vi "Main Page.vi"(8 "error in (no error)":errorcluster, 11 "Node Ptr":T7 format="%.0x") -> (0 "error out":errorcluster)   [LabVIEW 2015, in "Modbus Master System Explorer.lvlib"]
uses:
  Modbus Master System Explorer.lvlib
  <vilib>/NI Veristand/Custom Device API/Custom Device Item Ref.ctl
  Shared/Controls/Interface Type.ctl
  Shared/Controls/Parity.ctl
  Shared/Controls/Serial Type.ctl
  Shared/Controls/Flow Control.ctl
  SubVIs/Radix.ctl
  Shared/Constants.vi
  <vilib>/NI Veristand/Custom Device API/Set Item Property (U16).vi
  <vilib>/NI VeriStand/Custom Device API/Custom Device API.lvlib
  Shared/Modbus Master Shared.lvlib
panel:
  in  "WebBrowser":refnum<k7>(container)
  in  "Maximum Channels per Read":i32
  in  "Read Refresh Rate (ms)":i32
  in  "Export to Kepware Server":bool
  in  "Name":string
  in  "Master Settings Tabs":enum32{"TCP Master", "Serial Master"}(tab)
  in  "Timeout (ms)":i32
  in  "Address":string
  in  "Port":u16
  in  "Wire Mode":T1(ring)
  in  "Baud Rate":string(combo)
  in  "Radix":T2
  in  "Unit ID":u16
  out "Data Bits":u32=7
  in  "VISA resource name":refnum<visa-resource-name>
  in  "flow control (none)":T3 items=["None", "XON/XOFF", "RTS/CTS", "XON/XOFF & RTS/CTS", "DTR/DSR", "XON/XOFF & DTR/DSR"]
  in  "parity (even)":T4=2 items=["None", "Odd", "Even", "Mark", "Space"]
  in  "serial type":T5
  out "Stop Bits":u32
  in  "Interface Type":T6
  in  "Header":cluster{"Section Name":string}={"Section Name"="Modbus Master to Slave Settings"}
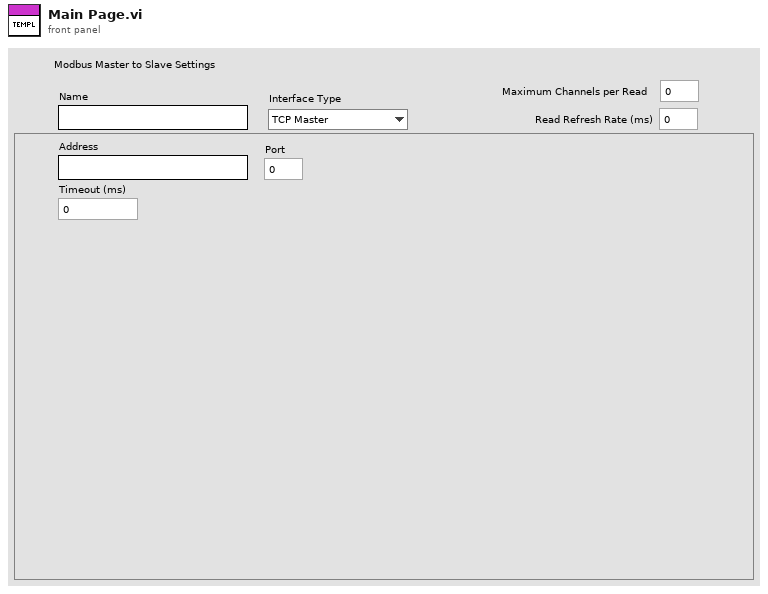
[diagram p1: front panel]
types:
  T1 = enum16{"Unknown", "RS485/Wire4", "RS485/Wire2-EchoDTR", "RS485/Wire2-CtrlDTR", "RS485/Wire2-Auto", "RS232/DTE", "RS232/DCE", "RS232/AUTO"}
  T2 = typedef "Modbus Master System Explorer.lvlib/Radix.ctl" = enum32{"Decimal", "Hexidecimal"}
  T3 = typedef "Modbus Master Shared.lvlib/Flow Control.ctl" = u16
  T4 = typedef "Modbus Master Shared.lvlib/Parity.ctl" = u16
  T5 = typedef "Modbus Master Shared.lvlib/Serial Type.ctl" = enum16{"RTU", "ASCII"}
  T6 = typedef "Modbus Master Shared.lvlib/Interface Type.ctl" = enum16{"TCP Master", "Serial Master", "TCP Slave", "Serial Slave"}
  T7 = typedef "Custom Device API.lvlib/Custom Device Item Ref.ctl" = u64
  T8 = typedef "Custom Device API.lvlib/Custom Device Commands.ctl" = enum16{"Default", "Item renamed", "Shutdown", "Dynamic button pressed"}
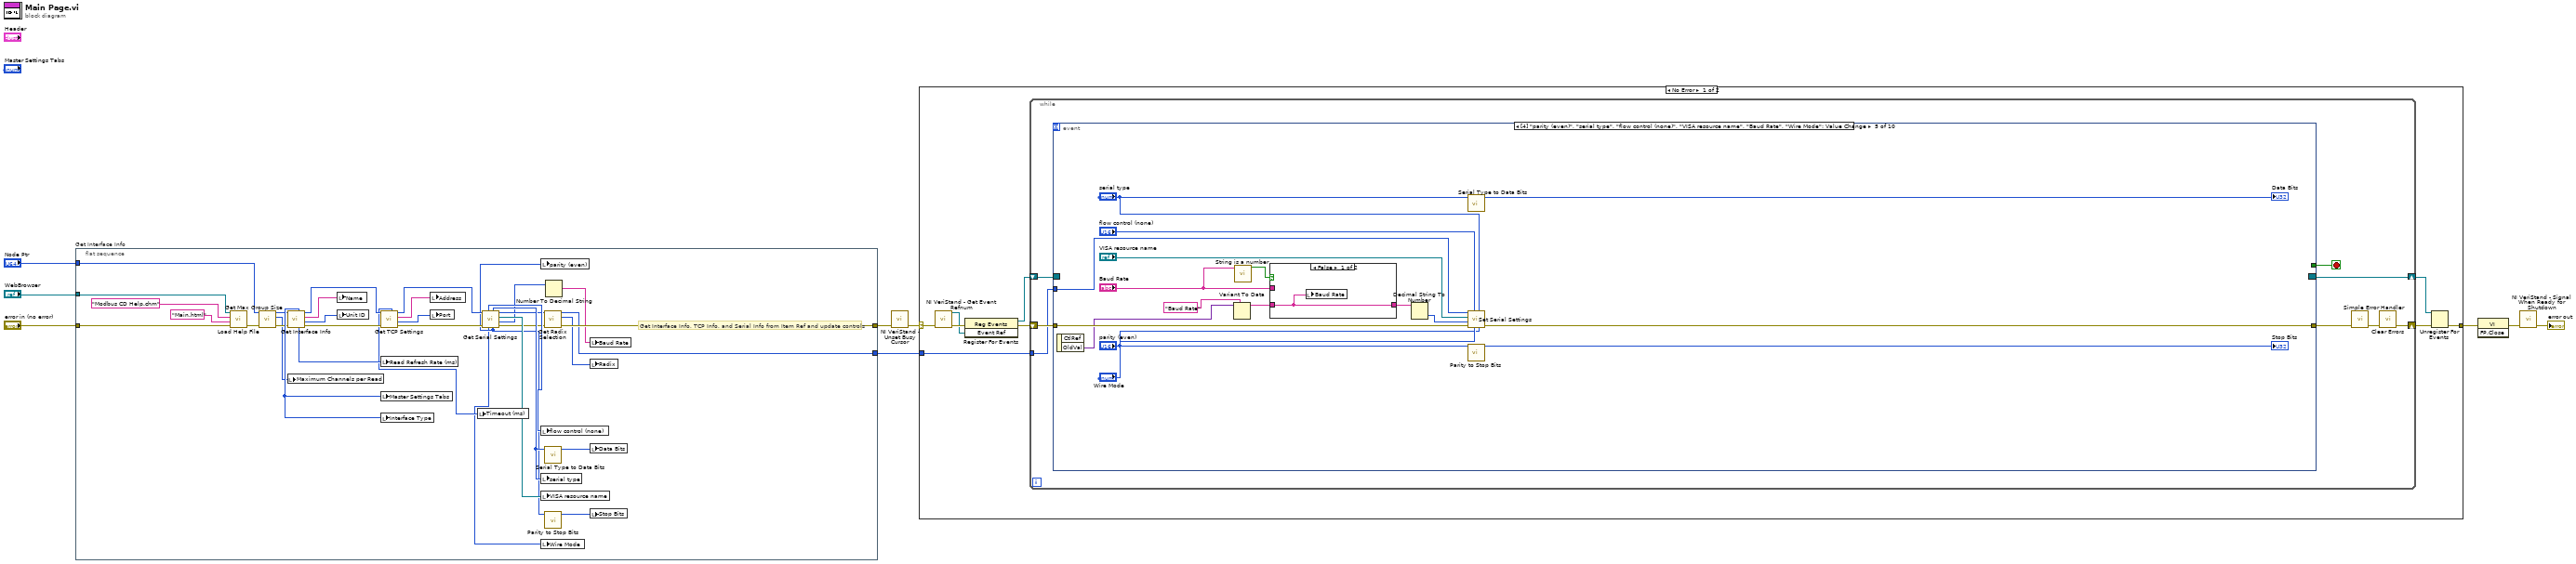
[diagram p0: block diagram]
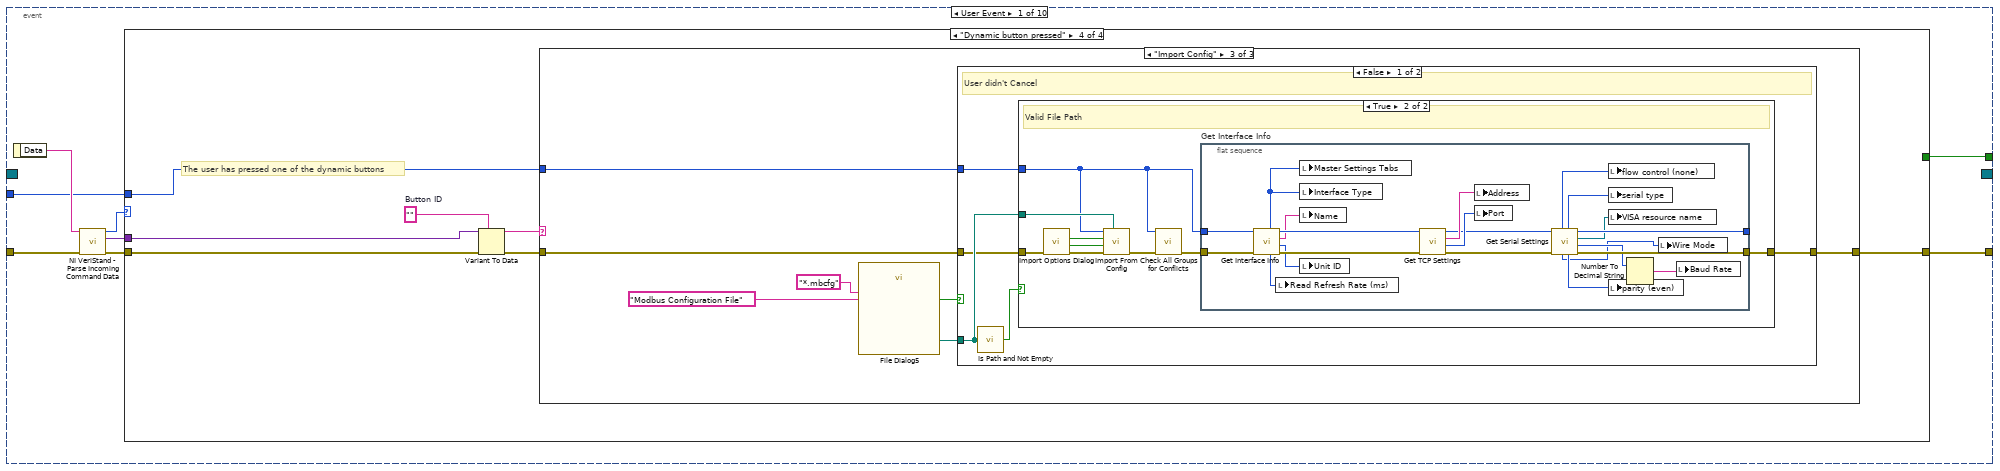
[diagram p2: hidden frame]
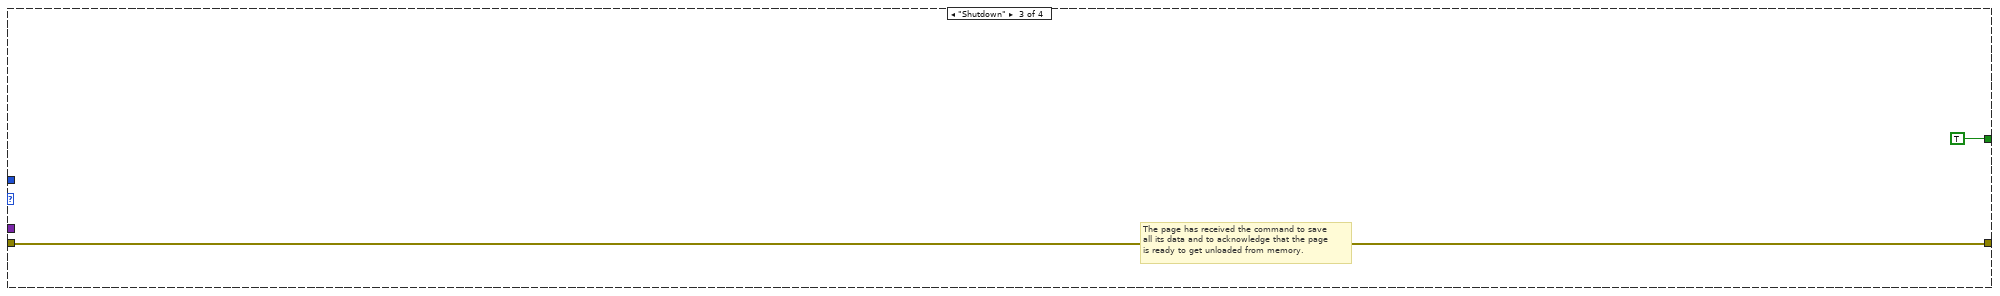
[diagram p5: hidden frame]
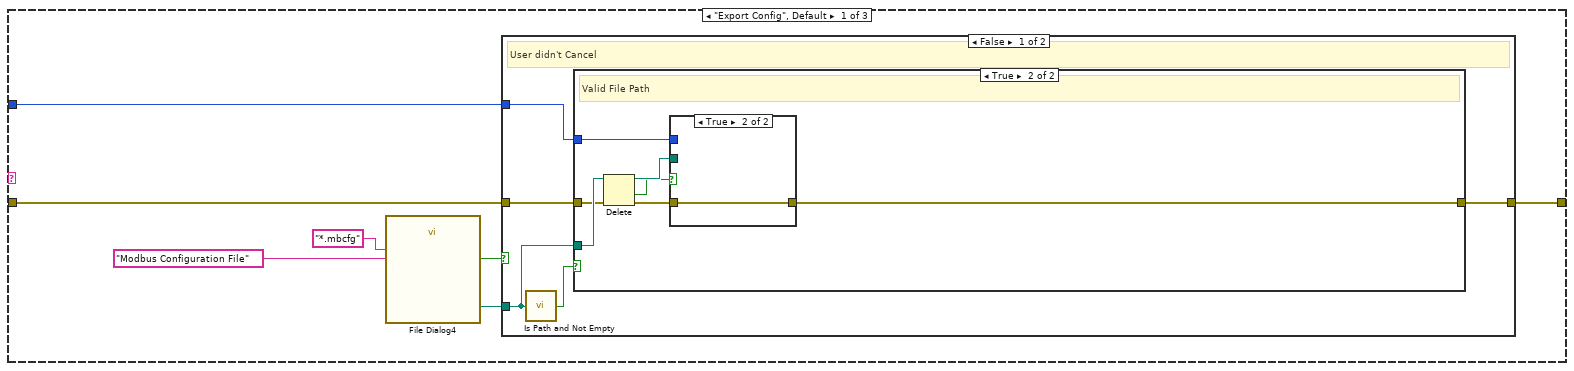
[diagram p6: hidden frame]
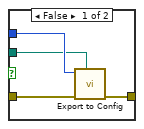
[diagram p8: hidden frame]
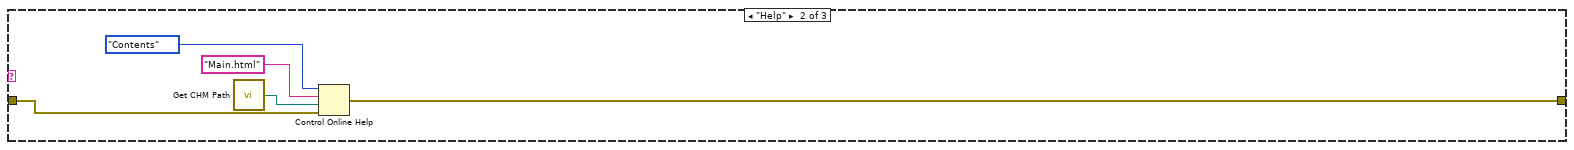
[diagram p10: hidden frame]
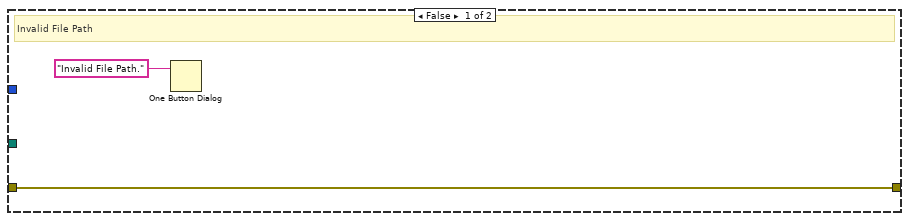
[diagram p11: hidden frame]
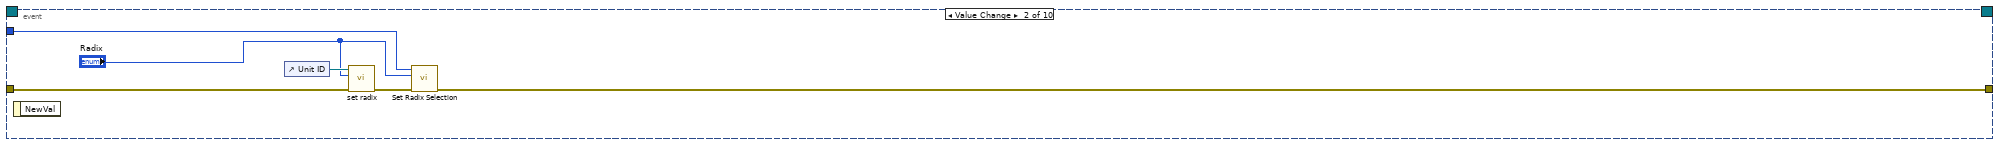
[diagram p13: hidden frame]
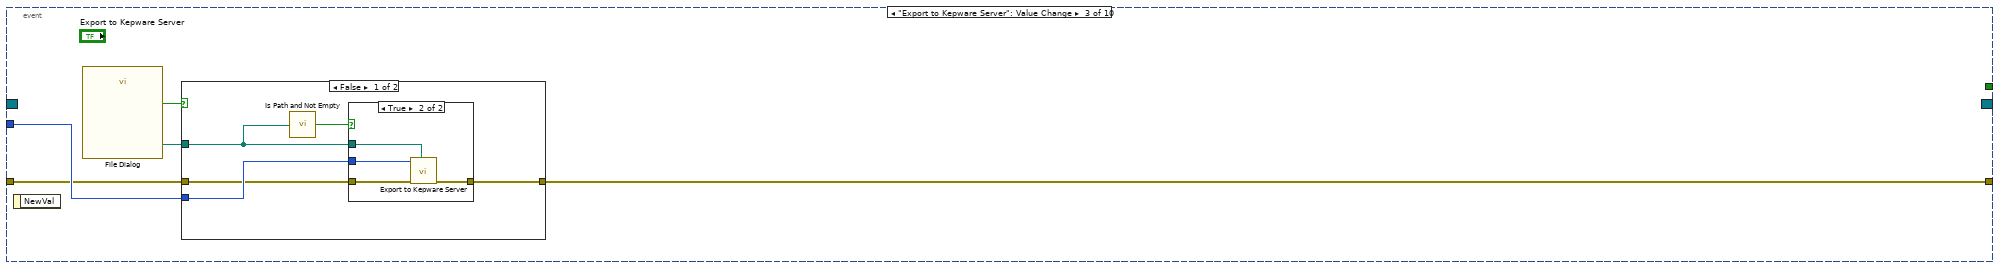
[diagram p14: hidden frame]
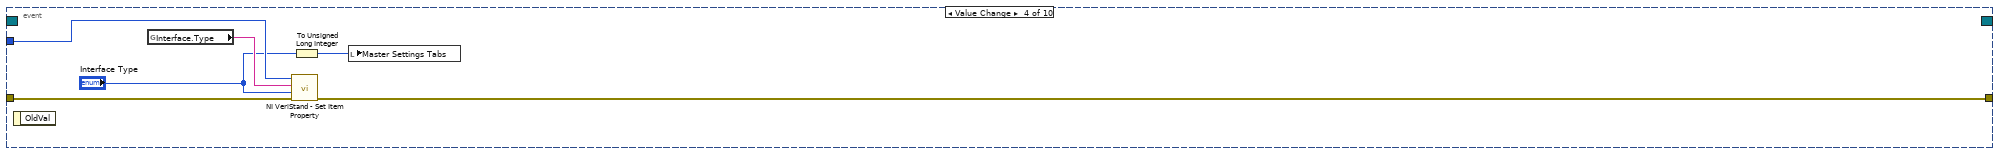
[diagram p17: hidden frame]
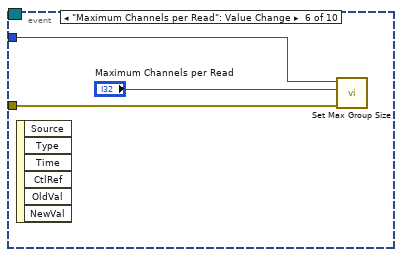
[diagram p19: hidden frame]
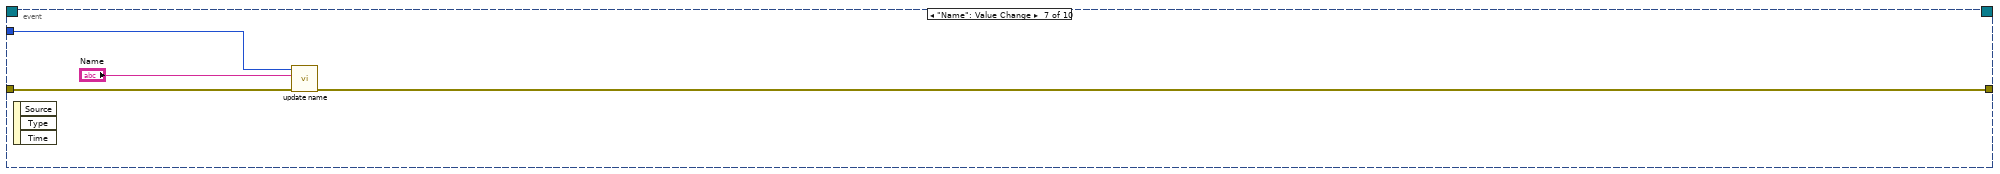
[diagram p20: hidden frame]
diagram:
  n1 = flat-sequence "Get Interface Info" {
    tunnel: "error in (no error)" -> [w12]
    tunnel: "Node Ptr" -> [w27]
    tunnel: [w21] -> w3
    tunnel: [w19] -> w2
    tunnel: "WebBrowser" -> [w15]
    frame #0 {
      # "Get Interface Info, TCP Info, and Serial Info from Item Ref and update controls"
      n2 = call "Load Help File.vi"("error in (no error)"=w12, "HTML File"="Main.html", "Main CHM File"="Modbus CD Help.chm", "SHDocVw.IWebBrowser2"=w15) -> ("error out"=w11:errorcluster)  [unwired: 7 in]
      n3 = call "Get Max Group Size.vi"("error in (no error)"=w11, "Item Ref in"=w27) -> ("error out"=w25:errorcluster, "Value"=w24:i32, "Item Ref out"=w26:T7)  [unwired: 7 in]
      n4 = call "Get Interface Info.vi"("error in (no error)"=w25, "Device Item Ref in"=w26) -> ("error out"=w36:errorcluster, "Unit ID"=w33:u16, "Name"=w34:string, "Item Ref out"=w37:T7, "Refresh Rate"=w32:i32, "Interface Type"=w35:T6)  [unwired: 4 in]
      n5 = local write "Maximum Channels per Read"(w24) -> ()
      n6 = local write "Name"(w34) -> ()
      n7 = local write "Unit ID"(w33) -> ()
      n8 = call "Get TCP Settings.vi"("error in (no error)"=w36, "Item Ref in"=w37) -> ("error out"=w41:errorcluster, "Port"=w42:u16, "Address"=w43:string, "Item Ref out"=w40:T7, "Timeout"=w23:i32)  [unwired: 5 in]
      n9 = local write "Read Refresh Rate (ms)"(w32) -> ()
      n10 = local write "Master Settings Tabs"(w35) -> ()
      n11 = local write "Interface Type"(w35) -> ()
      n12 = local write "Address"(w43) -> ()
      n13 = local write "Port"(w42) -> ()
      n14 = local write "Timeout (ms)"(w23) -> ()
      n15 = call "Get Serial Settings.vi"("error in (no error)"=w41, "Item Ref in"=w40) -> ("error out"=w22:errorcluster, "baud rate"=w17:u32, "VISA resource name"=w38:refnum<visa-resource-name>, "Item Ref out"=w20:T7, "parity (even)"=w29:T4, "serial type"=w30:T5, "Wire Mode"=w10:i16, "flow control (none)"=w39:T3)  [unwired: 2 in]
      n16 = local write "parity (even)"(w29) -> ()
      n17 = local write "flow control (none)"(w39) -> ()
      n18 = local write "serial type"(w30) -> ()
      n19 = local write "VISA resource name"(w38) -> ()
      n20 = local write "Wire Mode"(w10) -> ()
      n21 = call "Get Radix Selection.vi"("error in (no error)"=w22, "Item Ref in"=w20) -> ("error out"=w21:errorcluster, "Radix"=w18:T2, "Item Ref out"=w19:T7)  [unwired: 7 in]
      n22 = call "Serial Type to Data Bits.vi"("serial type"=w30) -> ("Data Bits"=w31:u32)  [unwired: 10 in]
      n23 = call "Parity to Stop Bits.vi"("parity"=w29) -> ("Stop Bits"=w28:u32)  [unwired: 10 in]
      n24 = Number To Decimal String(number=w17) -> (decimal integer string=w16:string)  [unwired: 1 in]
      n25 = local write "Baud Rate"(w16) -> ()
      n26 = local write "Radix"(w18) -> ()
      n27 = local write "Data Bits"(w31) -> ()
      n28 = local write "Stop Bits"(w28) -> ()
    }
  }
  n29 = call <vilib>:"NI VeriStand - Unset Busy Cursor.vi"("error in (no error)"=w3) -> ("error out"=w5:errorcluster)  [unwired: 10 out]
  n30 = case shown="No Error" w5 {
    selector: w5 -> [w44 w227]
    tunnel: [w49 w225] -> w9
    tunnel: w2 -> [w45 _]
    frame No Error {
      n31 = call <vilib>:"NI VeriStand - Get Event Refnum.vi"("error in (no error)"=w44) -> ("error out"=w52:errorcluster, "Event Ref"=w48:refnum<user-event>)  [unwired: 9 out]
      n32 = register-events(error in=w52, w48) -> (reference out=w46:refnum<event-registration>, error out=w47:errorcluster)  [unwired: 1 in]
      n33 = while {
        tunnel: w45 -> [w56]
        shift-right: [w53] -> w50
        shift-left: w47 -> [w59]
        shift-right: [w60] -> w51
        shift-left: w46 -> [w58]
        stop <- w57 stop-if-true
        n34 = event shown="[4] \"parity (even)\", \"serial type\", \"flow control (none)\", \"VISA resource name\", \"Baud Rate\", \"Wire Mode\": Value Change" {
          selector: w58 -> [_ _ _ _ _ _ _ _ _ _]
          dyn-events: [_ _ _ _ _ _ _ _ _ _] -> w60
          timeout: _ -> [_ _ _ _ _ _ _ _ _ _]
          tunnel: w59 -> [w68 w159 w163 w181 w198 w203 w207 w211 w217 w223]
          tunnel: [w64 _ _ _ _ _ _ _ _ _] -> w57
          tunnel: [w63 w157 w162 w178 w196 _ w206 w210 w216 w222] -> w55
          tunnel: w56 -> [w62 w161 w164 w182 w199 w205 w209 w212 w218 w224]
          event User Event {
            n35 = event-data() -> ("Data"=w67:string)  [unwired: 1 out]
            n36 = call <vilib>:"NI VeriStand - Parse Incoming Command Data.vi"("error in (no error)"=w68, "Incoming data"=w67) -> ("error out"=w66:errorcluster, "Outgoing data"=w61:variant, "Action"=w65:T8)  [unwired: 7 out]
            n37 = case shown="\"Dynamic button pressed\"" w65 {
              tunnel: w66 -> [w69 w70 w71 w79]
              tunnel: [_ _ TRUE _] -> w64
              tunnel: [w69 w70 w71 w73] -> w63
              tunnel: w62 -> [_ _ _ w75]
              tunnel: w61 -> [_ _ _ w78]
              frame "Default", Default {
              }
              frame "Item renamed" {
              }
              frame "Shutdown" {
                # "The page has received the command to save all its data and to acknowledge that the page is ready to get unloaded from memory."
              }
              frame "Dynamic button pressed" {
                w77 = ""  # Button ID
                # "The user has pressed one of the dynamic buttons"
                n38 = Variant To Data(error in=w79, type=w77, Variant=w78) -> (data=w76:string, error out=w74:errorcluster)
                n39 = case shown="\"Import Config\"" w76 {
                  tunnel: w75 -> [w84 _ w115]
                  tunnel: w74 -> [w83 w107 w114]
                  tunnel: [w82 w106 w113] -> w73
                  frame "Export Config", Default {
                    n40 = call "File Dialog4"("pattern (all files)"="*.mbcfg", "pattern label"="Modbus Configuration File") -> ("selected path"=w86:path, "cancelled"=w85:bool)  [unwired: 10 in, 2 out]
                    n41 = case shown="False" w85 {
                      tunnel: w86 -> [w90 _]
                      tunnel: w84 -> [w89 _]
                      tunnel: w83 -> [w88 w105]
                      tunnel: [w87 w105] -> w82
                      frame False {
                        # "User didn't Cancel"
                        n42 = call <vilib>:"Is Path and Not Empty.vi"("path"=w90) -> ("Is Path and Not Empty?"=w91:bool)  [unwired: 4 in]
                        n43 = case shown="True" w91 {
                          tunnel: w90 -> [_ w97]
                          tunnel: w89 -> [_ w98]
                          tunnel: w88 -> [w92 w94]
                          tunnel: [w92 w99] -> w87
                          frame False {
                          }
                          frame True {
                            # "Valid File Path"
                            n44 = Delete(path (use dialog)=w97, error in=w94) -> (deleted path=w96:path, cancelled=w95:bool, error out=w93:errorcluster)  [unwired: 3 in]
                            n45 = case shown="True" w95 {
                              tunnel: w93 -> [w103 w104]
                              tunnel: [w102 w104] -> w99
                              tunnel: w98 -> [w101 _]
                              tunnel: w96 -> [w100 _]
                              frame False {
                                n46 = call "Export to Config.vi"("selected path"=w100, "error in"=w103, "Device Ref in"=w101) -> ("error out"=w102:errorcluster)  [unwired: 8 in]
                              }
                              frame True {
                              }
                            }
                          }
                        }
                      }
                      frame True {
                      }
                    }
                  }
                  frame "Help" {
                    n47 = call "Get CHM Path.vi"() -> ("appended path"=w110:path)
                    n48 = Control Online Help(1:w107, 2:w110, 3:"Main.html" ("String to search for"), 4:enum16{"Contents", "Key", "Close"}."Contents" ("Operation")) -> (0:w106:errorcluster)
                  }
                  frame "Import Config" {
                    n49 = call "File Dialog5"("pattern (all files)"="*.mbcfg", "pattern label"="Modbus Configuration File") -> ("selected path"=w117:path, "cancelled"=w116:bool)  [unwired: 10 in, 2 out]
                    n50 = case shown="False" w116 {
                      tunnel: w117 -> [w121 _]
                      tunnel: w115 -> [w120 _]
                      tunnel: w114 -> [w119 w155]
                      tunnel: [w118 w155] -> w113
                      frame False {
                        # "User didn't Cancel"
                        n51 = call <vilib>:"Is Path and Not Empty.vi"("path"=w121) -> ("Is Path and Not Empty?"=w122:bool)  [unwired: 4 in]
                        n52 = case shown="True" w122 {
                          tunnel: w121 -> [_ w133]
                          tunnel: w120 -> [_ w131]
                          tunnel: w119 -> [w124 w128]
                          tunnel: [w124 w129] -> w118
                          frame False {
                            # "Invalid File Path"
                            n53 = One Button Dialog(message="Invalid File Path.") -> ()  [unwired: 1 in, 1 out]
                          }
                          frame True {
                            # "Valid File Path"
                            n54 = call "Import Options Dialog.vi"("error in (no error)"=w128) -> ("error out"=w127:errorcluster, "Overwrite Existing Channels?"=w125:bool, "Overwrite Device Settings?"=w126:bool)  [unwired: 8 in]
                            n55 = call "Import From Config.vi"("selected path"=w133, "error in"=w127, "Overwrite Existing Channels?"=w125, "Overwrite Device Settings?"=w126, "Device Ref in"=w131) -> ("error out"=w132:errorcluster)  [unwired: 6 in]
                            n56 = call "Check All Groups for Conflicts.vi"("error in (no error)"=w132, "Item Ref in"=w131) -> ("error out"=w130:errorcluster)  [unwired: 9 in]
                            n57 = flat-sequence "Get Interface Info" {
                              tunnel: w130 -> [w137]
                              tunnel: w131 -> [w138]
                              tunnel: [w151] -> w129
                              tunnel: [w149] -> _
                              frame #0 {
                                n58 = call "Get Interface Info.vi"("error in (no error)"=w137, "Device Item Ref in"=w138) -> ("error out"=w143:errorcluster, "Unit ID"=w140:u16, "Name"=w141:string, "Item Ref out"=w144:T7, "Refresh Rate"=w139:i32, "Interface Type"=w142:T6)  [unwired: 4 in]
                                n59 = local write "Read Refresh Rate (ms)"(w139) -> ()
                                n60 = local write "Master Settings Tabs"(w142) -> ()
                                n61 = local write "Interface Type"(w142) -> ()
                                n62 = local write "Name"(w141) -> ()
                                n63 = local write "Unit ID"(w140) -> ()
                                n64 = call "Get TCP Settings.vi"("error in (no error)"=w143, "Item Ref in"=w144) -> ("error out"=w152:errorcluster, "Port"=w153:u16, "Address"=w154:string, "Item Ref out"=w150:T7)  [unwired: 5 in, 1 out]
                                n65 = local write "Address"(w154) -> ()
                                n66 = local write "Port"(w153) -> ()
                                n67 = call "Get Serial Settings.vi"("error in (no error)"=w152, "Item Ref in"=w150) -> ("error out"=w151:errorcluster, "baud rate"=w136:u32, "VISA resource name"=w145:refnum<visa-resource-name>, "Item Ref out"=w149:T7, "parity (even)"=w148:T4, "serial type"=w147:T5, "Wire Mode"=w134:i16, "flow control (none)"=w146:T3)  [unwired: 2 in]
                                n68 = local write "flow control (none)"(w146) -> ()
                                n69 = local write "serial type"(w147) -> ()
                                n70 = local write "VISA resource name"(w145) -> ()
                                n71 = local write "parity (even)"(w148) -> ()
                                n72 = Number To Decimal String(number=w136) -> (decimal integer string=w135:string)  [unwired: 1 in]
                                n73 = local write "Wire Mode"(w134) -> ()
                                n74 = local write "Baud Rate"(w135) -> ()
                              }
                            }
                          }
                        }
                      }
                      frame True {
                        # "User Canecelled, do nothing"
                      }
                    }
                  }
                }
              }
            }
          }
          event Value Change {
            n75 = event-data() -> ()  [unwired: 2 out]
            n76 = control-ref of="Unit ID"() -> (w160:refnum<vi>)
            n77 = call "set radix.vi"("error in (no error)"=w159, "Radix"="Radix", "Digital in"=w160) -> ("error out"=w158:errorcluster)  [unwired: 8 in]
            n78 = call "Set Radix Selection.vi"("error in (no error)"=w158, "Radix"="Radix", "Item Ref in"=w161) -> ("error out"=w157:errorcluster)  [unwired: 7 in, 1 out]
          }
          event "Export to Kepware Server": Value Change {
            n79 = event-data() -> ()  [unwired: 2 out]
            n80 = call "File Dialog"() -> ("selected path"=w166:path, "cancelled"=w165:bool)  [unwired: 12 in, 2 out]
            n81 = case shown="False" w165 {
              tunnel: w166 -> [w170 _]
              tunnel: w164 -> [w169 _]
              tunnel: w163 -> [w168 w177]
              tunnel: [w167 w177] -> w162
              frame False {
                n82 = call <vilib>:"Is Path and Not Empty.vi"("path"=w170) -> ("Is Path and Not Empty?"=w171:bool)  [unwired: 4 in]
                n83 = case shown="True" w171 {
                  tunnel: w170 -> [_ w176]
                  tunnel: w169 -> [_ w175]
                  tunnel: w168 -> [w172 w174]
                  tunnel: [w172 w173] -> w167
                  frame False {
                  }
                  frame True {
                    n84 = call "Export to Kepware Server.vi"("selected path"=w176, "error in"=w174, "Device Ref in"=w175) -> ("error out"=w173:errorcluster)  [unwired: 8 in]
                  }
                }
              }
              frame True {
              }
            }
          }
          event Value Change {
            n85 = event-data() -> ()  [unwired: 2 out]
            n86 = global read "Constants.vi" "Interface.Type"() -> (w183:string)
            n87 = call-poly <vilib>:"NI VeriStand - Set Item Property.vi"("error in (no error)"=w181, "Value"="Interface Type", "Property Name"=w183, "Item Ref in"=w182) -> ("error out"=w178:errorcluster)  [unwired: 5 in, 2 out]
            n88 = To Unsigned Long Integer(number="Interface Type") -> (unsigned 32bit integer=w180:u32)
            n89 = local write "Master Settings Tabs"(w180) -> ()
          }
          event "VISA resource name", "Baud Rate", "Wire Mode": Value Change {
            n90 = event-data() -> ("OldVal"=w186:variant)  [unwired: 2 out]
            n91 = Variant To Data(type="Baud Rate" ("y"), Variant=w186) -> (data=w185:string)  [unwired: 1 in, 1 out]
            n92 = call "String is a number.vi"("Baud Rate"="Baud Rate") -> ("Boolean"=w189:bool)  [unwired: 10 in]
            n93 = case shown="False" w189 {
              tunnel: "Baud Rate" -> [_ w202]
              tunnel: [w201 w202] -> w187
              tunnel: w185 -> [w201 _]
              frame False {
                n94 = local write "Baud Rate"(w201) -> ()
              }
              frame True {
              }
            }
            n95 = Decimal String To Number(string=w187) -> (number=w193:i32)  [unwired: 2 in, 1 out]
            n96 = call "Serial Type to Data Bits.vi"("serial type"="serial type") -> ("Data Bits"=→"Data Bits":u32)  [unwired: 10 in]
            n97 = call "Set Serial Settings.vi"("Wire Mode"="Wire Mode", "serial type"="serial type", "parity (even)"="parity (even)", "flow control (none)"="flow control (none)", "error in (no error)"=w198, "baud rate"=w193, "VISA resource name"="VISA resource name", "Item Ref in"=w199) -> ("error out"=w196:errorcluster)  [unwired: 2 in, 1 out]
            n98 = call "Parity to Stop Bits.vi"("parity"="parity (even)") -> ("Stop Bits"=→"Stop Bits":u32)  [unwired: 10 in]
          }
          event "Maximum Channels per Read": Value Change {
            n99 = event-data() -> ()  [unwired: 7 out]
            n100 = call "Set Max Group Size.vi"("error in (no error)"=w203, "Value"="Maximum Channels per Read", "Item Ref in"=w205) -> ()  [unwired: 7 in, 2 out]
          }
          event "Name": Value Change {
            n101 = event-data() -> ()  [unwired: 4 out]
            n102 = call "update name.vi"("error in (no error)"=w207, "Desired Alias"="Name", "Parent Ref in"=w209) -> ("error out"=w206:errorcluster)  [unwired: 7 in, 1 out]
          }
          event "Unit ID": Value Change {
            n103 = event-data() -> ()  [unwired: 2 out]
            n104 = global read "Constants.vi" "Interface.UnitID"() -> (w214:string)
            n105 = call-poly <vilib>:"NI VeriStand - Set Item Property.vi"("error in (no error)"=w211, "Value"="Unit ID", "Property Name"=w214, "Item Ref in"=w212) -> ("error out"=w210:errorcluster)  [unwired: 5 in, 2 out]
          }
          event "Read Refresh Rate (ms)": Value Change {
            n106 = event-data() -> ()  [unwired: 5 out]
            n107 = call "Set Refresh Rate.vi"("error in (no error)"=w217, "Value"="Read Refresh Rate (ms)", "Item Ref in"=w218) -> ("error out"=w216:errorcluster)  [unwired: 7 in, 1 out]
          }
          event "Address", "Port", "Timeout (ms)": Value Change {
            n108 = event-data() -> ()  [unwired: 4 out]
            n109 = call "Set TCP Settings.vi"("Timeout"="Timeout (ms)", "error in (no error)"=w223, "Port"="Port", "Address"="Address", "Item Ref in"=w224) -> ("error out"=w222:errorcluster)  [unwired: 5 in, 1 out]
          }
        }
        n110 = call <vilib>:"Simple Error Handler.vi"("error in (no error)"=w55) -> ("error out"=w54:errorcluster)  [unwired: 1 in, 7 out]
        n111 = call <vilib>:"Clear Errors.vi"("error in (no error)"=w54) -> ("error out"=w53:errorcluster)  [unwired: 1 in, 5 out]
      }
      n112 = Unregister For Events(event registration refnum=w51, error in=w50) -> (error out=w49:errorcluster)
    }
    frame Error {
      n113 = call <vilib>:"Simple Error Handler.vi"("error in (no error)"=w227) -> ("error out"=w226:errorcluster)  [unwired: 1 in, 7 out]
      n114 = call <vilib>:"Clear Errors.vi"("error in (no error)"=w226) -> ("error out"=w225:errorcluster)  [unwired: 1 in, 5 out]
    }
  }
  n115 = invoke class="VI" method="FP.Close"(error in=w9) -> (error out=w8:errorcluster)  [unwired: 2 in, 2 out]
  n116 = call <vilib>:"NI VeriStand - Signal When Ready for Shutdown.vi"("error in (no error)"=w8) -> ("error out"=→"error out":errorcluster)  [unwired: 10 out]
